vi "6.vi"() -> ()   [LabVIEW 2020]
uses:
  <vilib>/numeric/Random Number (Range) DBL.vi
  0e066939-ad64-4988-be96-7d74cdbd5240.vi
  <vilib>/Comparison/Less/Less Functor/Less Functor.lvclass
panel:
  out "Waveform Graph 3":dbl[][](graph)
  in  "Array":dbl[][](array[numeric])
  out "Waveform Graph 2":dbl[](graph)
  out "Waveform Graph":dbl[](graph)
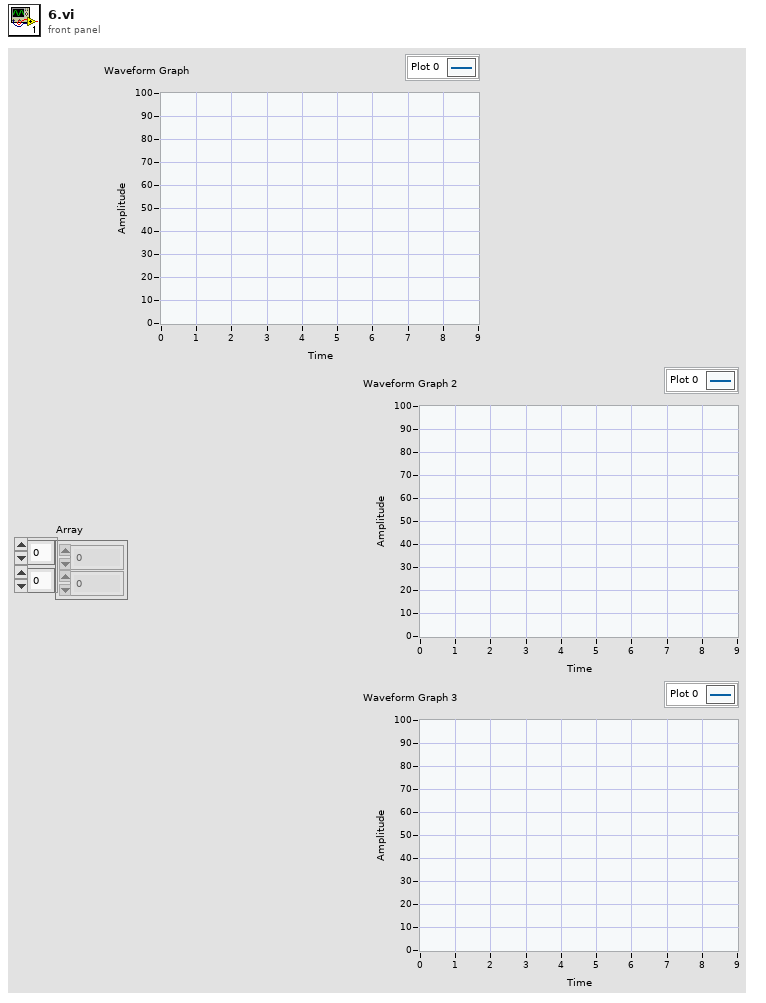
[diagram p1: front panel]
types:
  T1 = enum16{"open", "replace", "create", "open or create", "replace or create", "replace or create with confirmation"}
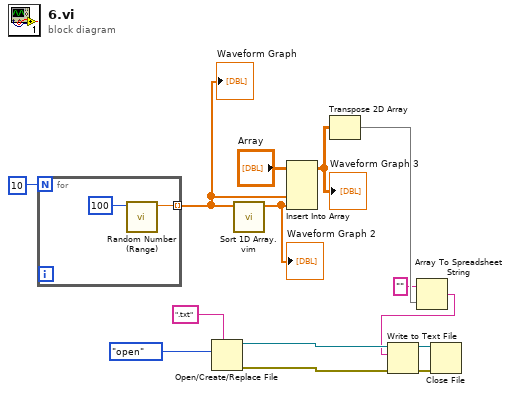
[diagram p0: block diagram]
diagram:
  n1 = for {
    N: 10 -> [_]
    tunnel: [w15] -> w6 mode=indexing
    n2 = call-poly <vilib>:"Random Number (Range).vi"("upper bound (100)"=u64 100) -> ("number"=w15:dbl)  [unwired: 10 in]
  }
  "Waveform Graph" <- w6
  n3 = Open/Create/Replace File(prompt=".txt" ("prompt (Choose or enter file path)"), operation (0:open)=T1."open") -> (refnum out=w12:refnum<file>, error out=w13:errorcluster)  [unwired: 4 in, 1 out]
  n4 = call "Sort 1D Array.vim"("unsorted array"=w6) -> ("sorted array"=w5:dbl[])  [unwired: 10 in]
  "Waveform Graph 2" <- w5
  n5 = Insert Into Array(array="Array", new element #1=w6, new element #2=w5) -> (w4:dbl[][])  [unwired: 2 in]
  "Waveform Graph 3" <- w4
  n6 = Transpose 2D Array(2D array=w4) -> (transposed array=w3:dbl[][])
  n7 = Array To Spreadsheet String(array=w3, 3:"" ("format string")) -> (spreadsheet string=w2:string)  [unwired: 1 in]
  n8 = Write to Text File(file (use dialog)=w12, text=w2, error in=w13) -> (refnum out=w9:refnum<file>, error out=w8:errorcluster)  [unwired: 1 in, 1 out]
  n9 = Close File(refnum=w9, error in=w8) -> ()  [unwired: 2 out]
